vi "Start.vi"(7 "Targets":string[](array[string]), 8 "error in (no error)":errorcluster, 11 "MSS Remote Actor in":refnum<class "MSS Remote Actor.lvclass">) -> (0 "error out":errorcluster, 3 "MSS Remote Actor out":refnum<class "MSS Remote Actor.lvclass">)   [LabVIEW 2023, in "MSS Remote Actor.lvlib" / "MSS Remote Actor.lvclass"]
uses:
  MSS Remote Actor.lvclass
  MSS Remote Actor.lvclass/MSS Remote Actor.ctl
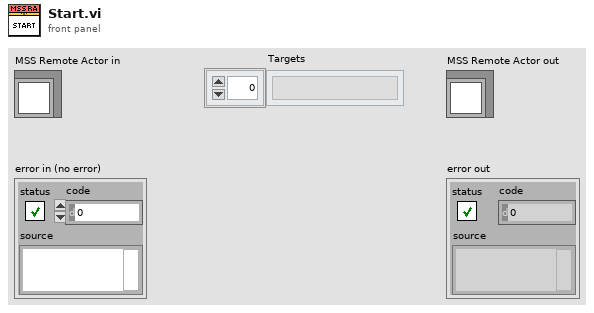
[diagram p1: front panel]
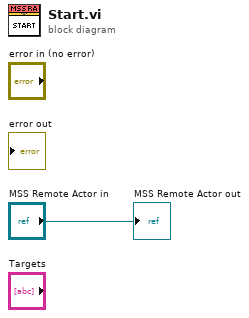
[diagram p0: block diagram]
diagram:
  "MSS Remote Actor out" <- "MSS Remote Actor in"
